vi "xmlToImage.vi"(8 "error in (no error)":errorcluster, 10 "xml":string, 11 "ImageStreamDecoder in":refnum<class "ImageStreamDecoder.lvclass">) -> (0 "error out":errorcluster, 2 "Image":T1, 3 "ImageStreamDecoder out":refnum<class "ImageStreamDecoder.lvclass">)   [LabVIEW 2011, in "Hardware.lvlib" / "HWControllers.lvlib" / "ImageStreamDecoder.lvclass"]
uses:
  ImageStreamDecoder.lvclass
  <vilib>/vision/Image Controls.llb/IMAQ Image.ctl
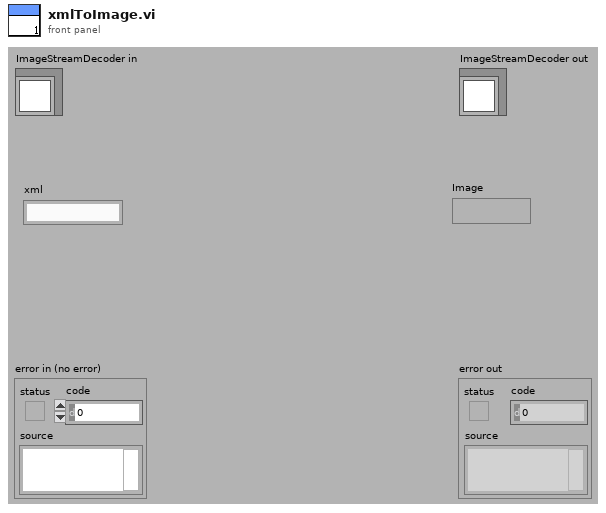
[diagram p1: front panel]
types:
  T1 = typedef "IMAQ Image.ctl" = refnum<image>
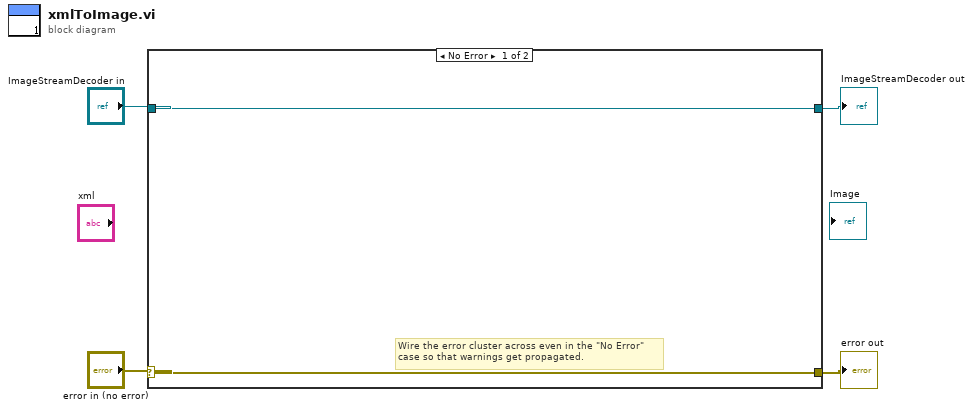
[diagram p0: block diagram]
diagram:
  n1 = case shown="No Error" "error in (no error)" {
    selector: "error in (no error)" -> [w5 w8]
    tunnel: [w5 w8] -> w3
    tunnel: [w6 w7] -> w1
    tunnel: "ImageStreamDecoder in" -> [w6 w7]
    frame No Error {
      # "Wire the error cluster across even in the \"No Error\"\ncase so that warnings get propagated."
    }
    frame Error {
    }
  }
  "error out" <- w3
  "ImageStreamDecoder out" <- w1
